vi "Main.vi"() -> ()   [LabVIEW 2020, in "Test App.lvclass"]
uses:
  Test App.lvclass
  build/ppl/Signal Generator.lvlibp/Signal Generator/Signal Generator.lvclass
  build/ppl/Scope.lvlibp/Scope/Scope.lvclass
  build/ppl/lv-hal.lvlibp/HAL Manager/HAL Manager.lvclass
  C:/dev/HAL Demo/build/ppl/lv-hal.lvlibp/Device/Device.lvclass
  build/ppl/lv-hal.lvlibp/Device/Device.lvclass
panel:
  out "Stop":bool
  out "Waveform Graph":dbl[](graph)
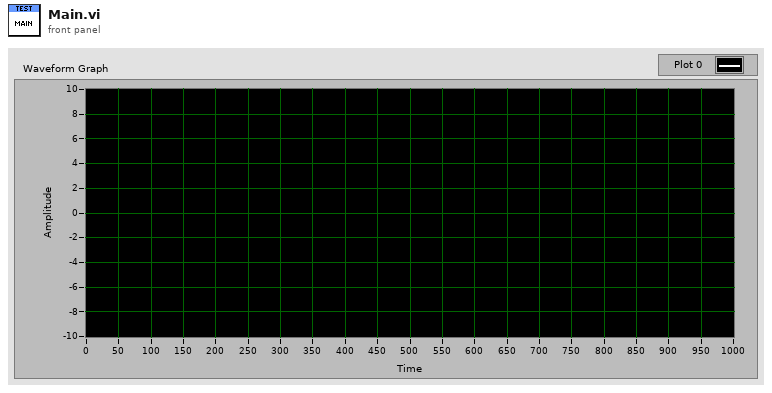
[diagram p1: front panel]
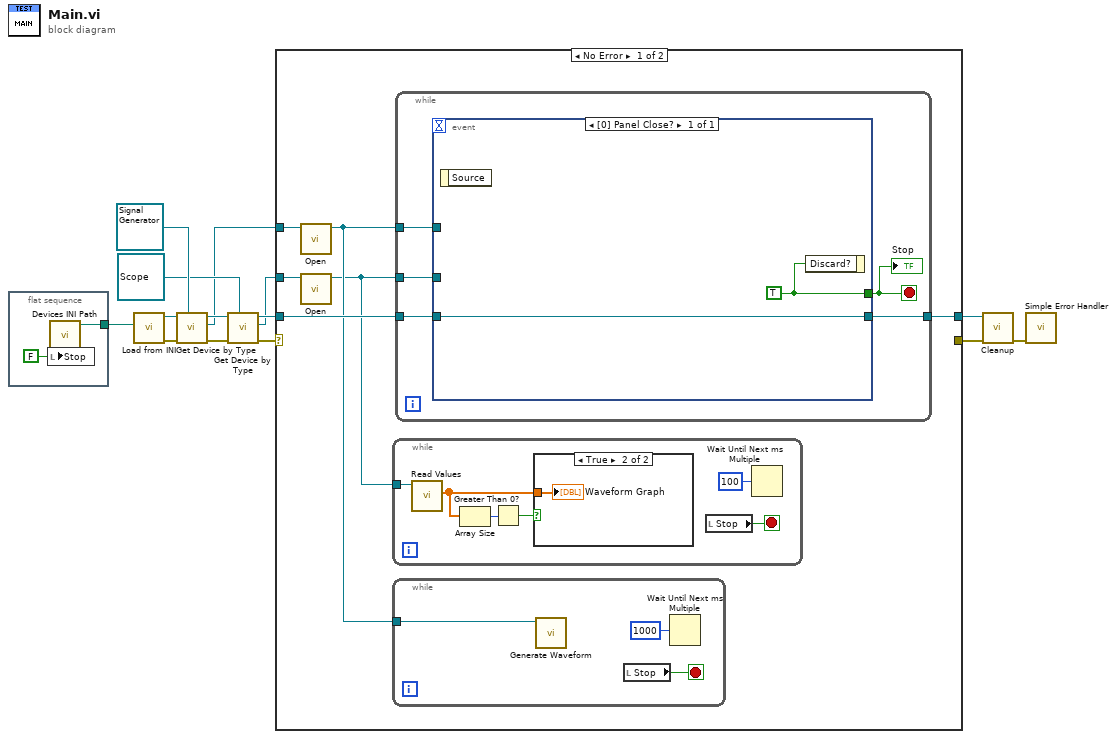
[diagram p0: block diagram]
diagram:
  n1 = flat-sequence {
    tunnel: [w16] -> w14
    frame #0 {
      n2 = local write "Stop"(FALSE ("Stop")) -> ()
      n3 = call "Devices INI Path.vi"() -> ("Devices INI Path"=w16:path)  [unwired: 11 in]
    }
  }
  n4 = call "Load from INI.vi"("INI Path"=w14) -> ("error out"=w6:errorcluster, "HAL Manager out"=w13:refnum<class "HAL Manager.lvclass">)  [unwired: 9 in]
  n5 = call "Get Device by Type.vi"("Device Type/Model"=refnum<class "Signal Generator.lvclass"> refnum ("Signal Generator.lvlibp:Signal Generator.lvclass"), "error in (no error)"=w6, "HAL Manager in"=w13) -> ("error out"=w5:errorcluster, "Device"=w7:refnum<class "Signal Generator.lvclass">, "HAL Manager out"=w10:refnum<class "HAL Manager.lvclass">)  [unwired: 6 in]
  n6 = call "Get Device by Type.vi"("Device Type/Model"=refnum<class "Scope.lvclass"> refnum ("Scope.lvlibp:Scope.lvclass"), "error in (no error)"=w5, "HAL Manager in"=w10) -> ("error out"=w4:errorcluster, "Device"=w8:refnum<class "Scope.lvclass">, "HAL Manager out"=w9:refnum<class "HAL Manager.lvclass">)  [unwired: 6 in]
  n7 = case shown="No Error" w4 {
    selector: w4 -> [_ w41]
    tunnel: w9 -> [w22 w40]
    tunnel: w8 -> [w18 _]
    tunnel: w7 -> [w20 _]
    tunnel: [_ w41] -> w2
    tunnel: [w21 w40] -> w3
    frame No Error {
      n8 = call "Open.vi"("Device in"=w20) -> ("Device out"=w19:refnum<class "Signal Generator.lvclass">)  [unwired: 9 in, 1 out]
      n9 = call "Open.vi"("Device in"=w18) -> ("Device out"=w17:refnum<class "Scope.lvclass">)  [unwired: 9 in, 1 out]
      n10 = while {
        tunnel: w17 -> [w26]
        stop <- w27 stop-if-true
        n11 = call-dynamic "Read Values.vi"("Scope in"=w26) -> ("Values"=w23:dbl[])  [unwired: 8 in, 2 out]
        n12 = Array Size(array=w23) -> (size(s)=w25:i32)
        n13 = Greater Than 0?(x=w25) -> (x > 0?=w24:bool)
        n14 = case shown="True" w24 {
          tunnel: w23 -> [_ w29]
          frame False {
          }
          frame True {
            "Waveform Graph" <- w29
          }
        }
        n15 = local read "Stop"() -> (w27:bool)
        n16 = Wait Until Next ms Multiple(millisecond multiple=u32 100) -> ()  [unwired: 1 out]
      }
      n17 = while {
        tunnel: w19 -> [w39]
        stop <- w37 stop-if-true
        n18 = call-dynamic "Generate Waveform.vi"("Signal Generator in"=w39) -> ()  [unwired: 9 in, 2 out]
        n19 = local read "Stop"() -> (w37:bool)
        n20 = Wait Until Next ms Multiple(millisecond multiple=u32 1000) -> ()  [unwired: 1 out]
      }
      n21 = while {
        tunnel: w17 -> [w34]
        tunnel: w19 -> [w33]
        tunnel: w22 -> [w31]
        tunnel: [w30] -> w21
        stop <- w32 stop-if-true
        n22 = event shown="[0] Panel Close?" {
          selector: _ -> [_]
          dyn-events: _ -> [_]
          timeout: _ -> [_]
          tunnel: w34 -> [_]
          tunnel: w33 -> [_]
          tunnel: [w35] -> w32
          tunnel: w31 -> [w36]
          tunnel: [w36] -> w30
          event Panel Close? {
            w35 = TRUE
            n23 = event-data() -> ()  [unwired: 1 in, 1 out]
            n24 = event-data("Discard?"=w35) -> ()  [unwired: 1 in, 1 out]
          }
        }
        "Stop" <- w32
      }
    }
    frame Error {
    }
  }
  n25 = call "Cleanup.vi"("error in (no error)"=w2, "HAL Manager in"=w3) -> ("error out"=w1:errorcluster)  [unwired: 9 in]
  n26 = call <vilib>:"Simple Error Handler.vi"("error in (no error)"=w1) -> ()  [unwired: 4 in, 5 out]
